vi "Vacuum Test - Step 4.vi"(7 "Step":i32, 8 "error in":errorcluster, 9 "Test Results In":T9, 10 "PAS In":T8 caption="Gas", 11 "Test Configuration":T1) -> (0 "error out":errorcluster, 1 "Test Results Out":T9, 2 "PAS Out":T8 caption="Gas", 3 "Test Configuration Out":T1)   [LabVIEW 2015]
uses:
  CAN Communication/PAS/Typedefs/Session Handle.ctl
  CAN Communication/PAS/PAS.lvclass
  Controls/Test Results.ctl
  Controls/Step Result.ctl
  Controls/Test Configuration.ctl
  Controls/Vacuum Test.ctl
  Controls/Test Timing.ctl
  Controls/Vaccum Thresholds.ctl
  Controls/Helium Test.ctl
  Controls/Helium Thresholds.ctl
  Controls/Functional Test.ctl
  CAN Communication/PAS/Typedefs/Valves.ctl
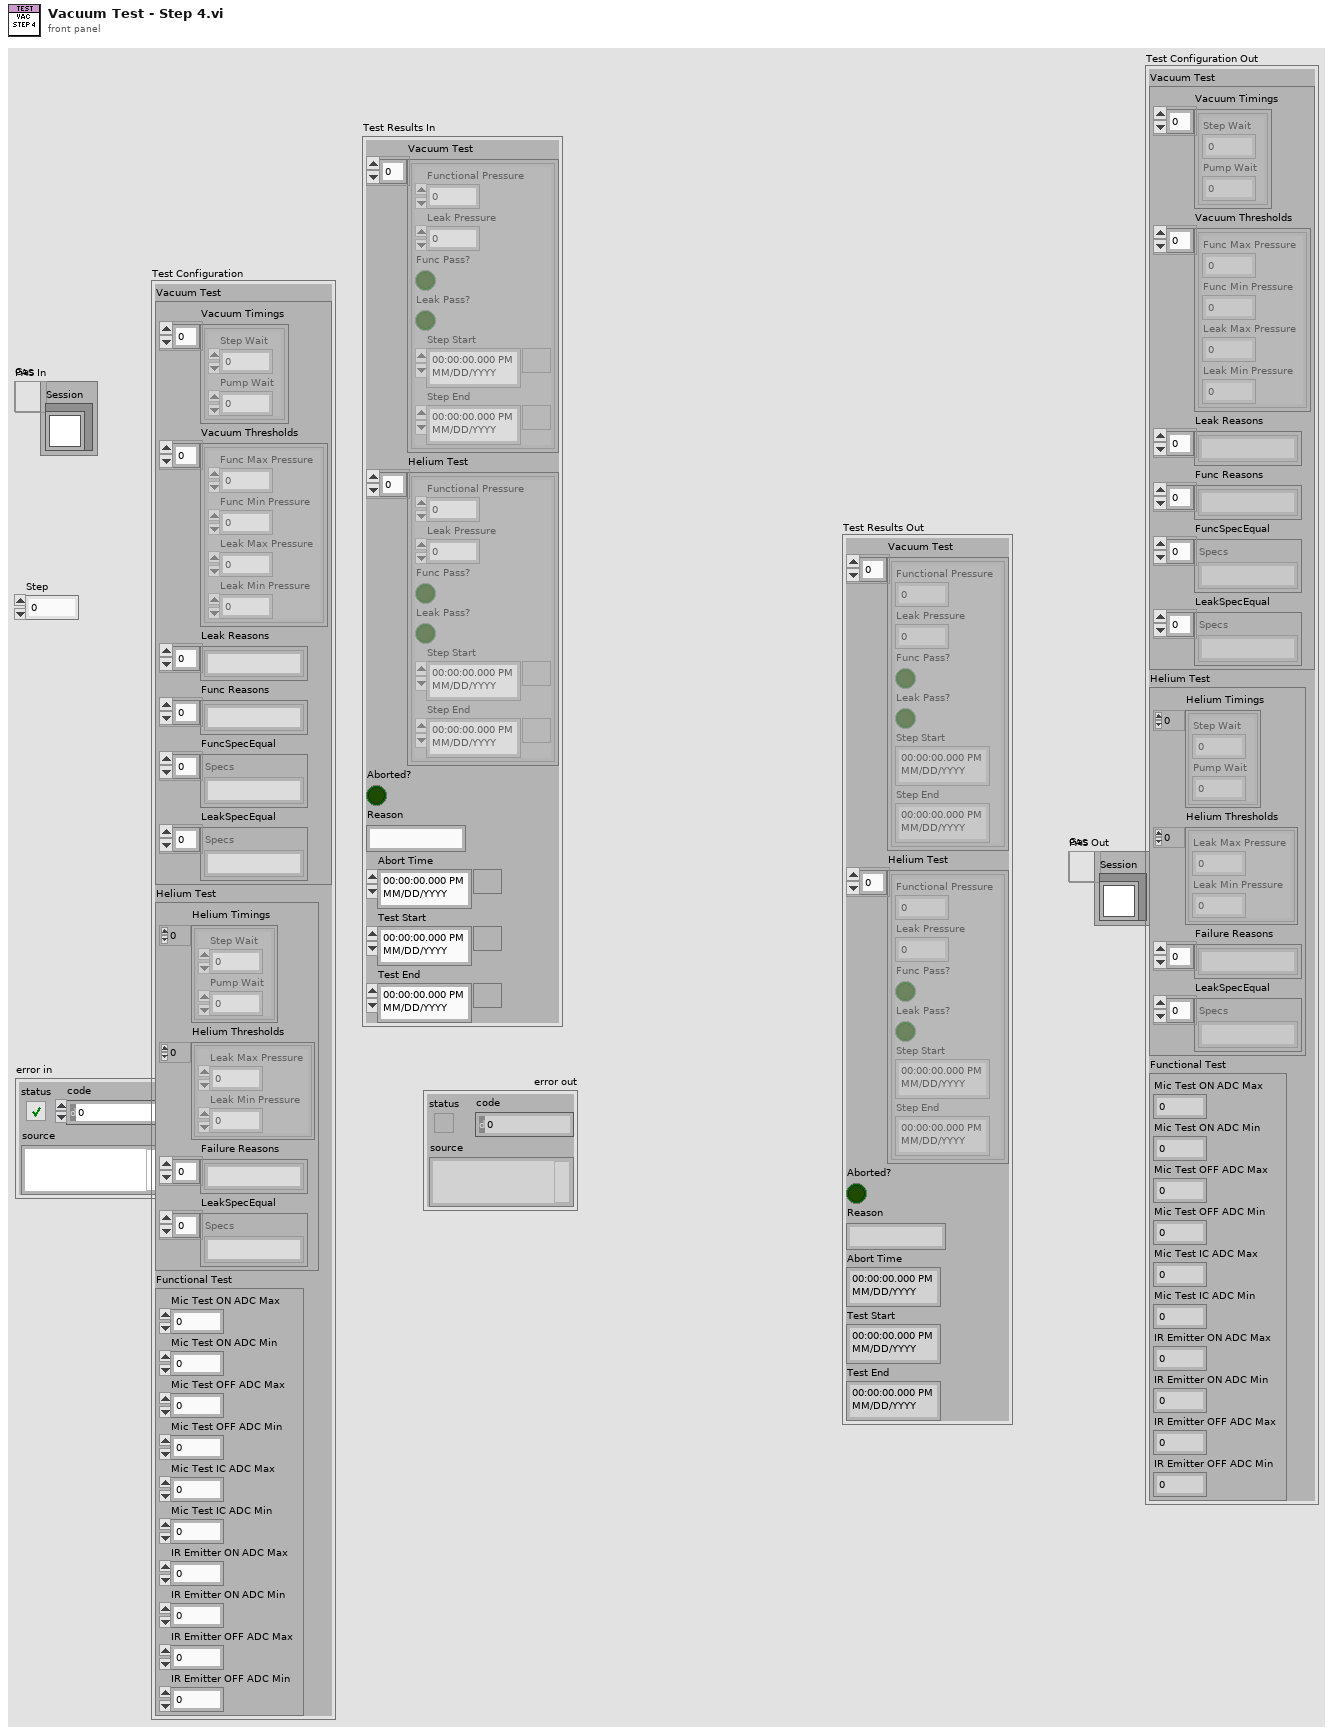
[diagram p1: front panel]
types:
  T1 = typedef "Test Configuration.ctl" = cluster{"Vacuum Test":T2, "Helium Test":T5, "Functional Test":T7}
  T2 = typedef "Vacuum Test.ctl" = cluster{"Vacuum Timings":T3[], "Vacuum Thresholds":T4[], "Leak Reasons":string[], "Func Reasons":string[], "FuncSpecEqual":string[], "LeakSpecEqual":string[]}
  T3 = typedef "Test Timing.ctl" = cluster{"Step Wait":dbl, "Pump Wait":dbl}
  T4 = typedef "Vaccum Thresholds.ctl" = cluster{"Func Max Pressure":dbl, "Func Min Pressure":dbl, "Leak Max Pressure":dbl, "Leak Min Pressure":dbl}
  T5 = typedef "Helium Test.ctl" = cluster{"Helium Timings":T3[], "Helium Thresholds":T6[], "Failure Reasons":string[], "LeakSpecEqual":string[]}
  T6 = typedef "Helium Thresholds.ctl" = cluster{"Leak Max Pressure":dbl, "Leak Min Pressure":dbl}
  T7 = typedef "Functional Test.ctl" = cluster{"Mic Test ON ADC Max":dbl, "Mic Test ON ADC Min":dbl, "Mic Test OFF ADC Max":dbl, "Mic Test OFF ADC Min":dbl, "Mic Test IC ADC Max":dbl, "Mic Test IC ADC Min":dbl, "IR Emitter ON ADC Max":dbl, "IR Emitter ON ADC Min":dbl, "IR Emitter OFF ADC Max":dbl, "IR Emitter OFF ADC Min":dbl}
  T8 = typedef "PAS.lvclass/Session Handle.ctl" = refnum<data-value>
  T9 = typedef "Test Results.ctl" = cluster{"Vacuum Test":T10[], "Helium Test":T10[], "Aborted?":bool, "Reason":string, "Abort Time":timestamp, "Test Start":timestamp, "Test End":timestamp}
  T10 = typedef "Step Result.ctl" = cluster{"Functional Pressure":dbl, "Leak Pressure":dbl, "Func Pass?":bool, "Leak Pass?":bool, "Step Start":timestamp, "Step End":timestamp}
  T11 = typedef "PAS.lvclass/Valves.ctl" = u16
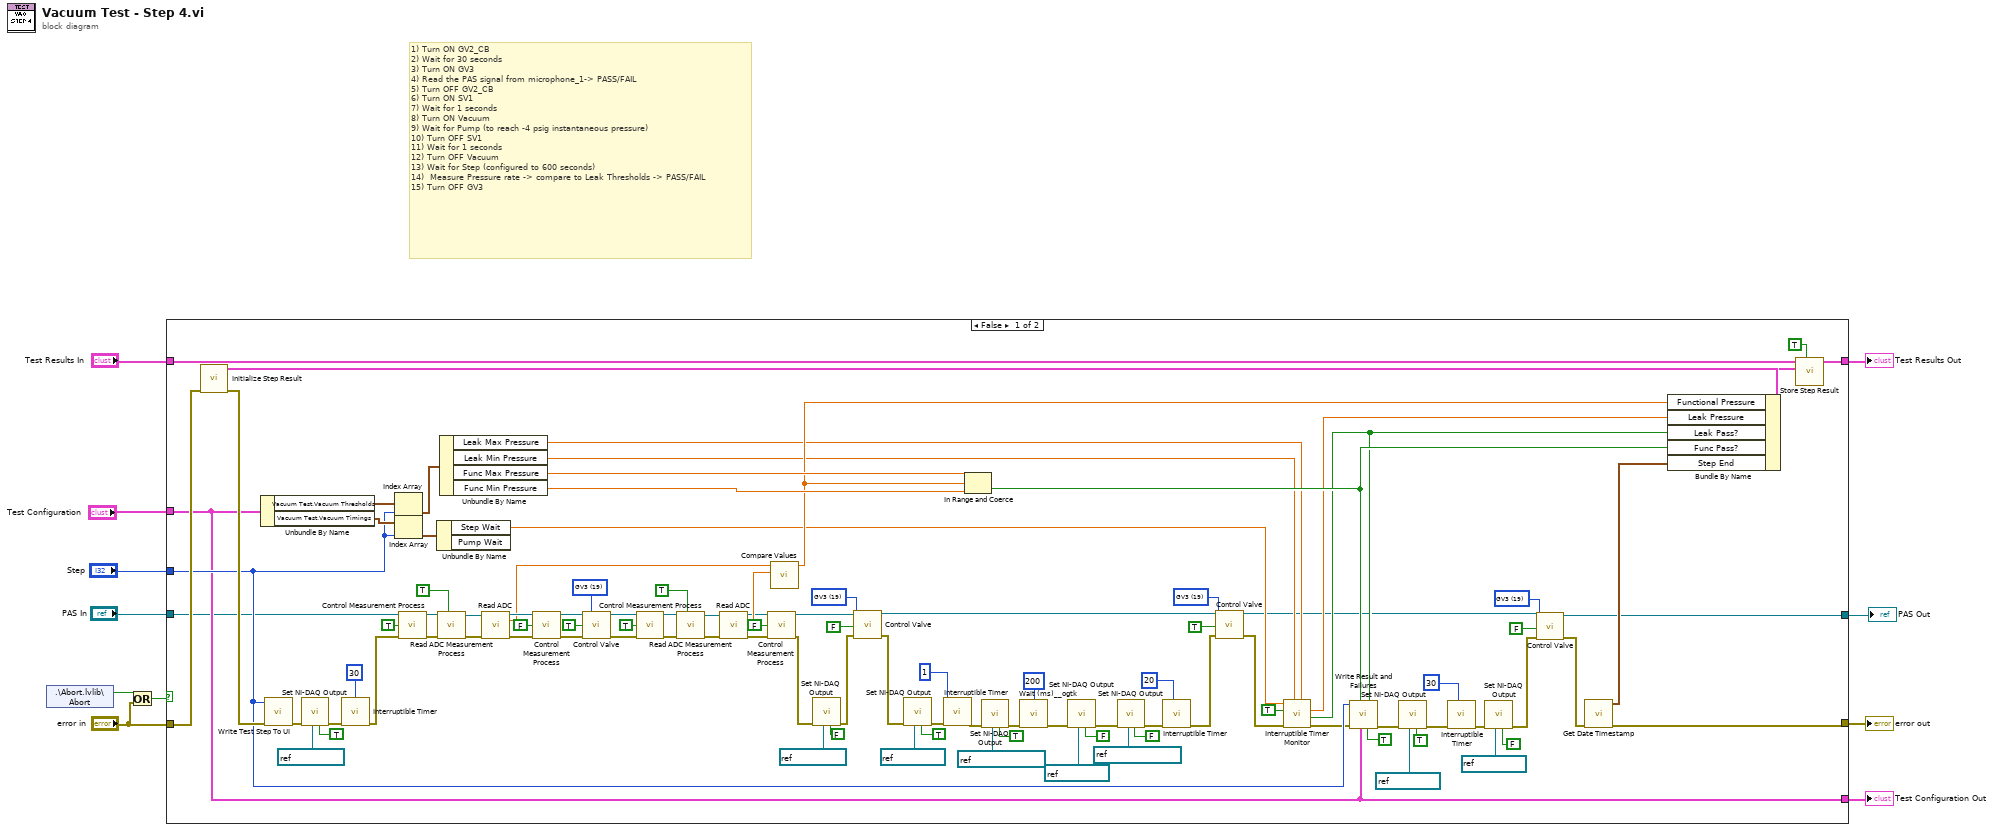
[diagram p0: block diagram]
diagram:
  # "1) Turn ON GV2_CB\n2) Wait for 30 seconds\n3) Turn ON GV3\n4) Read the PAS signal from microphone_1-> PASS/FAIL\n5) Turn OFF GV2_CB\n6) Turn ON SV1\n7) Wait for 1 seconds\n8) Turn ON Vacuum\n9) Wait for Pump (to reach -4 psig instantaneous pressure)\n10) Turn OFF SV1\n11) Wait for 1 seconds\n12) Turn OFF Vacuum\n13) Wait for Step (configured to 600 seconds)\n14)  Measure Pressure rate -> compare to Leak Thresholds -> PASS/FAIL\n15) Turn OFF GV3"
  n1 = shared-variable ".\\Abort.lvlib\\Abort"() -> (w10:bool)  [unwired: 1 in, 1 out]
  n2 = Or(x=w10, y="error in") -> (x .or. y?=w9:bool)
  n3 = case shown="False" w9 {
    tunnel: "error in" -> [w115 w118]
    tunnel: "Test Results In" -> [w112 w119]
    tunnel: [w113 w119] -> w7
    tunnel: [w13 w118] -> w6
    tunnel: "Test Configuration" -> [w93 w117]
    tunnel: "Step" -> [w103 _]
    tunnel: [w93 w117] -> w1
    tunnel: [w84 w116] -> w3
    tunnel: "PAS In" -> [w81 w116]
    frame False {
      w20 = T11 19 items=["GV1"=17, "GV2"=18, "GV3"=19, "GV4"=20] ("Valves")
      w28 = T11 19 items=["GV1"=17, "GV2"=18, "GV3"=19, "GV4"=20] ("Valves")
      w74 = T11 19 items=["GV1"=17, "GV2"=18, "GV3"=19, "GV4"=20] ("Valves")
      w86 = T11 19 items=["GV1"=17, "GV2"=18, "GV3"=19, "GV4"=20] ("Valves")
      n4 = call "Initialize Step Result.vi"("error in (no error)"=w115) -> ("error out"=w114:errorcluster, "New Step Result"=w111:T10)  [unwired: 8 in, 1 out]
      n5 = Unbundle By Name(w93) -> ("Vacuum Test.Vacuum Thresholds"=w108:T4[], "Vacuum Test.Vacuum Timings"=w107:T3[])
      n6 = call "Write Test Step To UI.vi"("error in (no error)"=w114, "Step"=w103) -> ("error out"=w101:errorcluster)  [unwired: 9 in]
      n7 = call "Set NI-DAQ Output.vi"("State"=TRUE, "Channel"=refnum<k21> "GV2_PAS", "error in (no error)"=w101) -> ("error out"=w100:errorcluster)  [unwired: 8 in]
      n8 = call "Interruptible Timer.vi"("error in (no error)"=w100, "Wait (s)"=30) -> ("error out"=w80:errorcluster)  [unwired: 7 in, 2 out]
      n9 = Index Array(array=w108, index=w103) -> (element=w104:T4)
      n10 = Index Array(array=w107, index=w103) -> (element=w106:T3)
      n11 = call "Control Measurement Process.vi"("Session Handle in"=w81, "Start?"=TRUE, "error in (no error)"=w80) -> ("Session Handle out"=w59:T8, "error out"=w58:errorcluster)  [unwired: 9 in, 2 out]
      n12 = Unbundle By Name(w106) -> ("Step Wait"=w45:dbl)  [unwired: 1 out]
      n13 = call "Read ADC Measurement Process.vi"("Measurement Started?"=TRUE, "error in (no error)"=w58, "Session Handle in"=w59) -> ("error out"=w56:errorcluster, "Session Handle out"=w57:T8)  [unwired: 6 in, 1 out]
      n14 = Unbundle By Name(w104) -> ("Leak Max Pressure"=w42:dbl, "Leak Min Pressure"=w43:dbl, "Func Max Pressure"=w67:dbl, "Func Min Pressure"=w66:dbl)
      n15 = call "Read ADC.vi"("Session Handle in"=w57, "error in (no error)"=w56) -> ("Session Handle out"=w79:T8, "ADC"=w69:dbl, "error out"=w78:errorcluster)  [unwired: 10 in, 1 out]
      n16 = call "Control Measurement Process.vi"("Session Handle in"=w79, "Start?"=FALSE, "error in (no error)"=w78) -> ("Session Handle out"=w76:T8, "error out"=w75:errorcluster)  [unwired: 9 in, 2 out]
      n17 = call "Control Valve.vi"("Session Handle in"=w76, "Valves"=w74, "Energize?"=TRUE, "error in (no error)"=w75) -> ("Session Handle out"=w71:T8, "error out"=w70:errorcluster)  [unwired: 8 in, 2 out]
      n18 = call "Control Measurement Process.vi"("Session Handle in"=w71, "Start?"=TRUE, "error in (no error)"=w70) -> ("Session Handle out"=w54:T8, "error out"=w53:errorcluster)  [unwired: 9 in, 2 out]
      n19 = call "Read ADC Measurement Process.vi"("Measurement Started?"=TRUE, "error in (no error)"=w53, "Session Handle in"=w54) -> ("error out"=w52:errorcluster, "Session Handle out"=w51:T8)  [unwired: 6 in, 1 out]
      n20 = call "Read ADC.vi"("Session Handle in"=w51, "error in (no error)"=w52) -> ("Session Handle out"=w64:T8, "ADC"=w68:dbl, "error out"=w63:errorcluster)  [unwired: 10 in, 1 out]
      n21 = call "Control Measurement Process.vi"("Session Handle in"=w64, "Start?"=FALSE, "error in (no error)"=w63) -> ("Session Handle out"=w26:T8, "error out"=w62:errorcluster)  [unwired: 9 in, 2 out]
      n22 = call "Compare Values.vi"("P2"=w68, "P1"=w69) -> ("Abs Diff"=w60:dbl)  [unwired: 9 in]
      n23 = call "Set NI-DAQ Output.vi"("State"=FALSE, "Channel"=refnum<k21> "GV2_PAS", "error in (no error)"=w62) -> ("error out"=w25:errorcluster)  [unwired: 8 in]
      n24 = call "Control Valve.vi"("Session Handle in"=w26, "Valves"=w28, "Energize?"=FALSE, "error in (no error)"=w25) -> ("Session Handle out"=w19:T8, "error out"=w24:errorcluster)  [unwired: 8 in, 2 out]
      n25 = call "Set NI-DAQ Output.vi"("State"=TRUE, "Channel"=refnum<k21> "SV1_PAS", "error in (no error)"=w24) -> ("error out"=w31:errorcluster)  [unwired: 8 in]
      n26 = call "Interruptible Timer.vi"("error in (no error)"=w31, "Wait (s)"=1) -> ("error out"=w30:errorcluster)  [unwired: 7 in, 2 out]
      n27 = In Range and Coerce(upper limit=w67, x=w60, lower limit=w66) -> (In Range?=w65:bool)  [unwired: 1 out]
      n28 = call "Set NI-DAQ Output.vi"("State"=TRUE, "Channel"=refnum<k21> "Vacuum_PAS", "error in (no error)"=w30) -> ("error out"=w48:errorcluster)  [unwired: 8 in]
      n29 = call <userlib>:"Wait (ms)__ogtk.vi"("error in (no error)"=w48, "milliseconds to wait"=u32 200) -> ("error out"=w47:errorcluster)  [unwired: 8 in, 1 out]
      n30 = call "Set NI-DAQ Output.vi"("State"=FALSE, "Channel"=refnum<k21> "SV1_PAS", "error in (no error)"=w47) -> ("error out"=w49:errorcluster)  [unwired: 8 in]
      n31 = call "Set NI-DAQ Output.vi"("State"=FALSE, "Channel"=refnum<k21> "Vacuum_PAS", "error in (no error)"=w49) -> ("error out"=w23:errorcluster)  [unwired: 8 in]
      n32 = call "Interruptible Timer.vi"("error in (no error)"=w23, "Wait (s)"=20) -> ("error out"=w17:errorcluster)  [unwired: 7 in, 2 out]
      n33 = call "Control Valve.vi"("Session Handle in"=w19, "Valves"=w20, "Energize?"=TRUE, "error in (no error)"=w17) -> ("Session Handle out"=w18:T8, "error out"=w16:errorcluster)  [unwired: 8 in, 2 out]
      n34 = call "Interruptible Timer Monitor.vi"("Max"=w42, "Min"=w43, "error in (no error)"=w16, "Update UI?"=TRUE, "Wait (s)"=w45) -> ("error out"=w15:errorcluster, "In Range?"=w40:bool, "Leak Rate"=w41:dbl)  [unwired: 3 in, 1 out]
      n35 = call "Write Result and Failures.vi"("Vacuum?"=TRUE, "Leak"=w40, "Test Configuration"=w93, "Func"=w65, "error in (no error)"=w15, "Step"=w103) -> ("error out"=w14:errorcluster)  [unwired: 5 in]
      n36 = call "Set NI-DAQ Output.vi"("State"=TRUE, "Channel"=refnum<k21> "SV1_PAS", "error in (no error)"=w14) -> ("error out"=w37:errorcluster)  [unwired: 8 in]
      n37 = call "Interruptible Timer.vi"("error in (no error)"=w37, "Wait (s)"=30) -> ("error out"=w35:errorcluster)  [unwired: 7 in, 2 out]
      n38 = call "Set NI-DAQ Output.vi"("State"=FALSE, "Channel"=refnum<k21> "SV1_PAS", "error in (no error)"=w35) -> ("error out"=w32:errorcluster)  [unwired: 8 in]
      n39 = call "Control Valve.vi"("Session Handle in"=w18, "Valves"=w86, "Energize?"=FALSE, "error in (no error)"=w32) -> ("Session Handle out"=w84:T8, "error out"=w83:errorcluster)  [unwired: 8 in, 2 out]
      n40 = call "Get Date Timestamp.vi"("error in (no error)"=w83) -> ("error out"=w13:errorcluster, "current time"=w109:timestamp)  [unwired: 9 in]
      n41 = Bundle By Name(cluster=w111, "Functional Pressure"=w60, "Leak Pressure"=w41, "Leak Pass?"=w40, "Func Pass?"=w65, "Step End"=w109) -> (w110:T10)
      n42 = call "Store Step Result.vi"("Vacuum?"=TRUE, "Step Result"=w110, "Test Results In"=w112) -> ("Test Results Out"=w113:T9)  [unwired: 8 in]
    }
    frame True {
    }
  }
  "error out" <- w6
  "Test Results Out" <- w7
  "PAS Out" <- w3
  "Test Configuration Out" <- w1
